vi "add application firewall rule.vi"   [LabVIEW 2016]
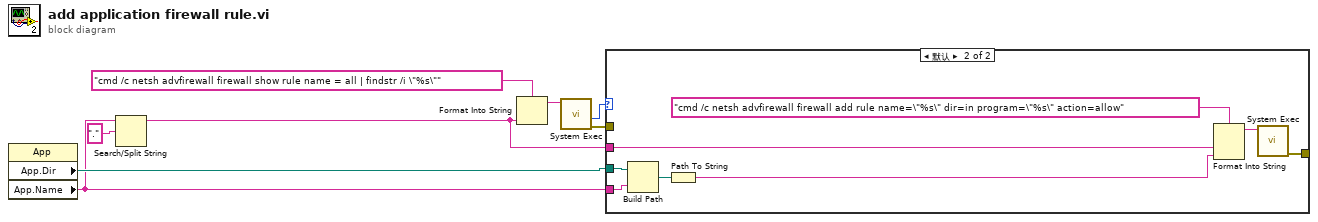
[diagram p0: block diagram]
diagram:
  n1 = property class="App"() -> ("App.Dir"=w8:path, "App.Name"=w6:string)  [unwired: 2 in, 2 out]
  n2 = Search/Split String(string=w6, search string/char (-)="." ("搜索字符串/字符(-)")) -> (substring before match=w5:string)  [unwired: 1 in, 2 out]
  n3 = Format Into String(format string="cmd /c netsh advfirewall firewall show rule name = all | findstr /i \"%s\"" ("command line"), w5) -> (resulting string=w4:string)  [unwired: 2 in, 1 out]
  n4 = call <vilib>:"System Exec.vi"("command line"=w4) -> ("error out"=w2:errorcluster, "return code"=w3:i32)  [unwired: 7 in, 2 out]
  n5 = case shown="默认" w3 {
    tunnel: w8 -> [_ w16]
    tunnel: w6 -> [_ w12]
    tunnel: w5 -> [_ w10]
    tunnel: w2 -> [_ _]
    tunnel: [_ w9] -> _
    frame 0 {
    }
    frame Default {
      n6 = Build Path(base path=w16, name or relative path=w12) -> (appended path=w15:path)
      n7 = Path To String(path=w15) -> (string=w13:string)
      n8 = Format Into String(format string="cmd /c netsh advfirewall firewall add rule name=\"%s\" dir=in program=\"%s\" action=allow" ("command line"), w10, w13) -> (resulting string=w11:string)  [unwired: 2 in, 1 out]
      n9 = call <vilib>:"System Exec.vi"("command line"=w11) -> ("error out"=w9:errorcluster)  [unwired: 7 in, 3 out]
    }
  }
